vi "GetEventInterface.vi"(8 "error in (no error)":errorcluster, 11 "Window in":refnum<class "Window.lvclass">) -> (0 "error out":errorcluster, 2 "Event Interface":refnum<class "WindowEventInterface.lvclass">, 3 "Window out":refnum<class "Window.lvclass">)   [LabVIEW 2020, in "GLF.lvlib" / "Window.lvclass"]
uses:
  Window.lvclass
  WindowEventInterface/WindowEventInterface.lvclass
  Window.lvclass/Window.ctl
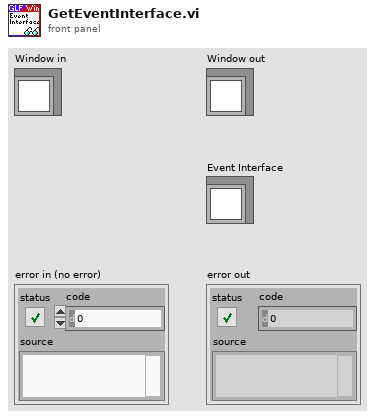
[diagram p1: front panel]
types:
  T1 = typedef "GLF.lvlib/Window.lvclass/DVR--cluster.ctl" = cluster{"SDL_Window *":T2, "Window ID":T3, "SDL_Renderer *":T4, "Event Interface":refnum<class "WindowEventInterface.lvclass">}
  T2 = typedef "SDL3.lvlib/Video.lvlib/SDL_Window--pointer.ctl" = i64
  T3 = typedef "SDL3.lvlib/Video.lvlib/WindowID--integer.ctl" = u32
  T4 = typedef "SDL3.lvlib/Render.lvlib/SDL_Renderer--pointer.ctl" = i64
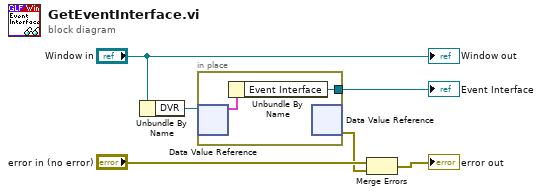
[diagram p0: block diagram]
diagram:
  n1 = Unbundle By Name("Window in") -> ("DVR"=w3:refnum<data-value>)
  n2 = in-place {
    in-place-border: [w8] -> w1
    n3 = in-place-dvr #1(w3) -> (w7:T1)  [unwired: 1 out]
    n4 = Unbundle By Name(w7) -> ("Event Interface"=w8:refnum<class "WindowEventInterface.lvclass">)
    n5 = in-place-dvr #1() -> (w2:errorcluster)  [unwired: 1 in, 1 out]
  }
  "Event Interface" <- w1
  n6 = Merge Errors("error in (no error)", w2) -> (→"error out":errorcluster)
  "Window out" <- "Window in"
